vi "Write Dbl File v1.vi"(5 "data":sgl[](array[numeric]), 6 "error in":errorcluster, 7 "axis lengths":T1, 8 "pixel numbers":T2, 9 "Path":path) -> (0 "error out":errorcluster)   [LabVIEW 2014]
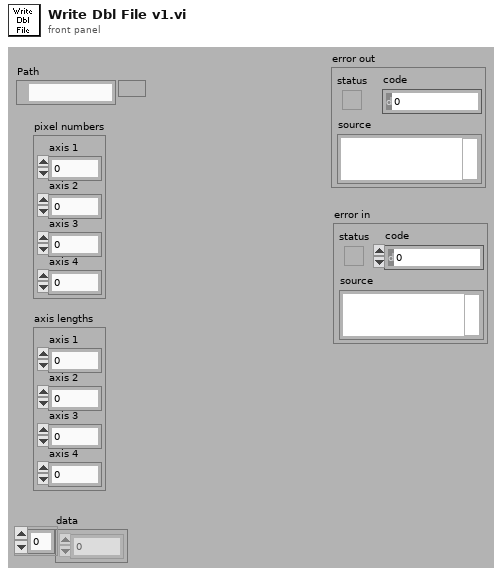
[diagram p1: front panel]
types:
  T1 = cluster{"axis 1":dbl, "axis 2":dbl, "axis 3":dbl, "axis 4":dbl}
  T2 = cluster{"axis 1":u16, "axis 2":u16, "axis 3":u16, "axis 4":u16}
  T3 = enum16{"big-endian, network order", "native, host order", "little-endian"}
  T4 = enum16{"deny read/write", "deny write-only", "deny none"}
  T5 = enum16{"open", "replace", "create", "open or create", "replace or create", "replace or create with confirmation"}
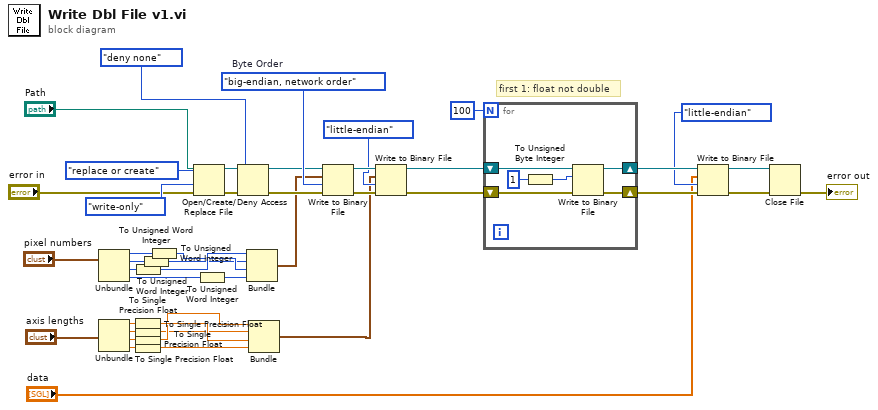
[diagram p0: block diagram]
diagram:
  w36 = T3."big-endian, network order"  # Byte Order
  # "first 1: float not double"
  n1 = Unbundle("pixel numbers") -> ("axis 1"=w28:u16, "axis 2"=w27:u16, "axis 3"=w26:u16, "axis 4"=w25:u16)
  n2 = Unbundle("axis lengths") -> ("axis 1"=w20:dbl, "axis 2"=w19:dbl, "axis 3"=w18:dbl, "axis 4"=w17:dbl)
  n3 = To Unsigned Word Integer(number=w26) -> (unsigned 16bit integer=w23:u16)
  n4 = To Single Precision Float(number=w20) -> (single precision float=w14:sgl)
  n5 = To Single Precision Float(number=w19) -> (single precision float=w12:sgl)
  n6 = To Single Precision Float(number=w18) -> (single precision float=w13:sgl)
  n7 = To Single Precision Float(number=w17) -> (single precision float=w15:sgl)
  n8 = To Unsigned Word Integer(number=w27) -> (unsigned 16bit integer=w21:u16)
  n9 = To Unsigned Word Integer(number=w28) -> (unsigned 16bit integer=w22:u16)
  n10 = Open/Create/Replace File(file path (use dialog)="Path", error in="error in", operation (0:open)=T5."replace or create", access (0:read/write)=enum16{"read/write", "read-only", "write-only"}."write-only") -> (refnum out=w41:refnum<file>, error out=w40:errorcluster)  [unwired: 3 out]
  n11 = To Unsigned Word Integer(number=w25) -> (unsigned 16bit integer=w24:u16)
  n12 = Deny Access(4:w40, 6:T4."deny none" ("deny mode (0:deny read/write)"), 7:w41) -> (0:w35:errorcluster, 3:w34:refnum<file>)
  n13 = Bundle(w23, w21, w22, w24) -> (w6:cluster{u16, u16, u16, u16})  [unwired: 1 out]
  n14 = Bundle(w13, w12, w14, w15) -> (w16:cluster{sgl, sgl, sgl, sgl})  [unwired: 1 out]
  n15 = Write to Binary File(file (use dialog)=w34, data=w6, error in=w35, 9:w36) -> (refnum out=w32:refnum<file>, error out=w33:errorcluster)  [unwired: 3 out]
  n16 = Write to Binary File(file (use dialog)=w32, data=w16, error in=w33, 9:T3."little-endian" ("byte order (0:big-endian, network order)")) -> (refnum out=w9:refnum<file>, error out=w10:errorcluster)  [unwired: 3 out]
  n17 = for {
    N: 100 -> [_]
    shift-right: [w47] -> w7
    shift-left: w9 -> [w49]
    shift-right: [w46] -> w8
    shift-left: w10 -> [w48]
    n18 = To Unsigned Byte Integer(number=u8 1) -> (unsigned 8bit integer=w45:u8)
    n19 = Write to Binary File(file (use dialog)=w49, data=w45, error in=w48) -> (refnum out=w47:refnum<file>, error out=w46:errorcluster)  [unwired: 1 in, 3 out]
  }
  n20 = Write to Binary File(file (use dialog)=w7, data="data", error in=w8, 9:T3."little-endian" ("byte order (0:big-endian, network order)")) -> (refnum out=w4:refnum<file>, error out=w3:errorcluster)  [unwired: 3 out]
  n21 = Close File(refnum=w4, error in=w3) -> (error out=→"error out":errorcluster)  [unwired: 1 out]
